vi "WPI_CameraOpen.vi"(8 "error in (no error)":errorcluster, 9 "Disallow Simulation":bool, 11 "Camera Address":string="192.168.0.90") -> (0 "error out":errorcluster, 3 "CameraDevRef":T1)   [LabVIEW 2017]
doc: "Opens a reference to the camera you specify. This reference can then be used with the other functions on the camera palette. If a reference to the camera is already open, this VI returns an error.\n\nThis software is licensed. Open the labview\\readme\\WPI Robotics Library Open Source License.txt file for more information."
uses:
  <vilib>/Rock Robotics/WPI/Camera/WPI_CameraRegistryActions.ctl
  <vilib>/robotics/Simulator/Engine/ctl/DeviceID.ctl
  <vilib>/robotics/Simulator/NI_Robotics_Simulator.lvlib
  <vilib>/Rock Robotics/WPI/Camera/WPI_CameraDevRef.ctl
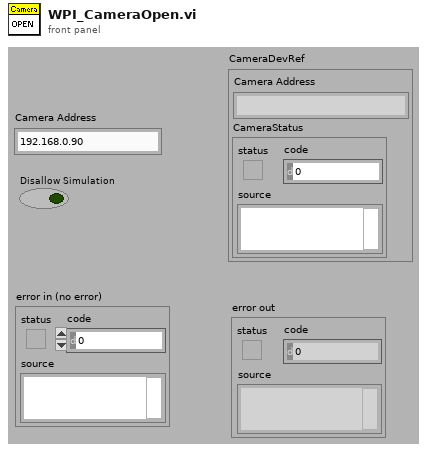
[diagram p1: front panel]
types:
  T1 = typedef "WPI_CameraDevRef.ctl" = cluster{"Camera Address":string, "CameraStatus":errorcluster}
  T2 = typedef "WPI_CameraRegistryActions.ctl" = enum16{"Open", "Close"}
  T3 = typedef "NI_Robotics_Simulator.lvlib/DeviceID.ctl" = cluster{"robot ID":string, "sensor/actuator ID":string}
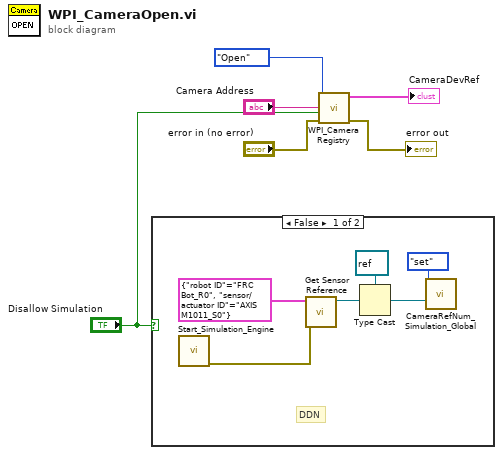
[diagram p0: block diagram]
diagram:
  n1 = case shown="False" "Disallow Simulation" {
    frame False {
      # "DDN"
      n2 = call <vilib>:"Start_Simulation_Engine.vi"() -> ("error out"=w7:errorcluster)  [unwired: 15 in]
      n3 = call <vilib>:"Get Sensor Reference.vi"("error in (no error)"=w7, "device ID"=T3 {"robot ID"="FRC Bot_R0", "sensor/actuator ID"="AXIS M1011_S0"} ("Device ID")) -> ("sensor ref"=w9:refnum<k20>)  [unwired: 8 in, 1 out]
      n4 = Type Cast(type=refnum<k20> refnum ("Accelerometer Out"), x=w9) -> (*(type *) &x=w11:refnum<k20>)
      n5 = call <vilib>:"CameraRefNum_Simulation_Global.vi"("menu"=enum16{"set", "get", "delete"}."set", "Axis M1011 Set"=w11) -> ()  [unwired: 12 in, 2 out]
    }
    frame True {
    }
  }
  n6 = call <vilib>:"WPI_Camera Registry.vi"("error in (no error)"="error in (no error)", 9:"Disallow Simulation", "Camera Address"="Camera Address", "Action"=WPI_CameraRegistryActions."Open" ("Enum")) -> ("error out"=→"error out":errorcluster, "CameraDevRef"=→"CameraDevRef":T1)  [unwired: 6 out]
